vi "구구단.vi"() -> ()   [LabVIEW 2014]
panel:
  in  "정지":bool
  in  "y":i32
  out "배열":i32[][](array[numeric])
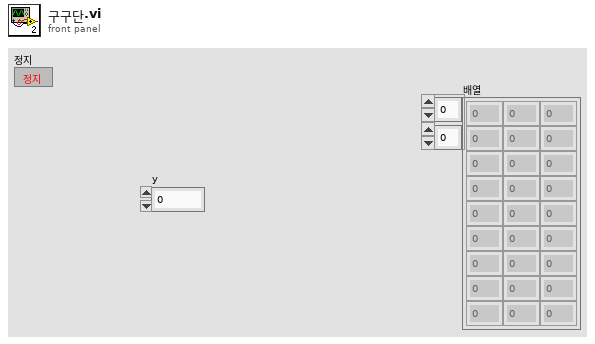
[diagram p1: front panel]
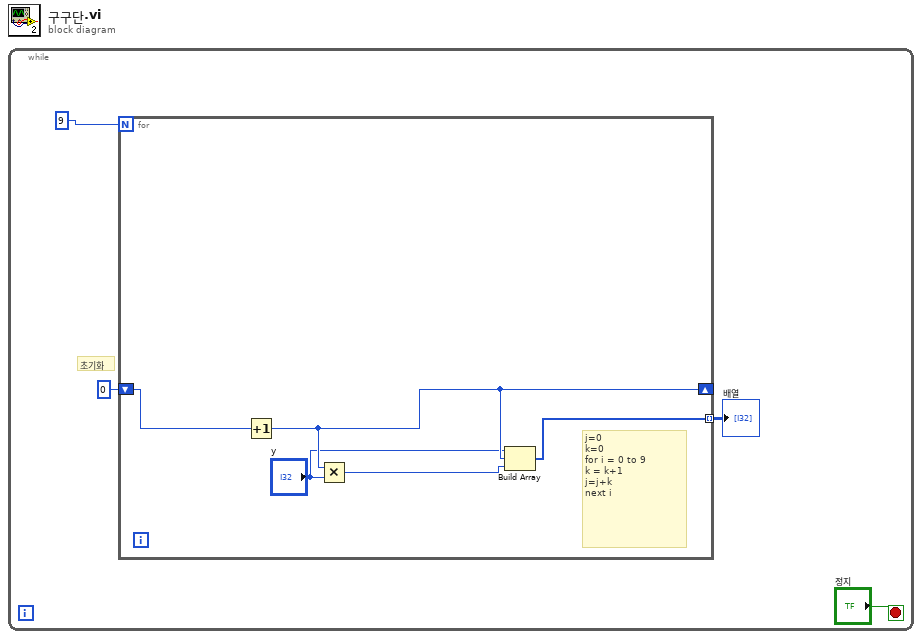
[diagram p0: block diagram]
diagram:
  n1 = while {
    stop <- "정지" stop-if-true
    # "초기화"
    n2 = for {
      N: 9 -> [_]
      shift-right: [w7] -> _
      shift-left: 0 -> [w9]
      tunnel: [w6] -> w2 mode=indexing
      # "j=0\nk=0\nfor i = 0 to 9\nk = k+1\nj=j+k\nnext i"
      n3 = Increment(x=w9) -> (x+1=w7:i32)
      n4 = Multiply(x=w7, y="y") -> (x*y=w8:i32)
      n5 = Build Array("y", w7, w8) -> (w6:i32[])
    }
    "배열" <- w2
  }
